vi "AC Voltage Configure.vi"(7 "ChannelList":string, 8 "error in (no error)":errorcluster {"code" format="%.0x"}, 9 "Resolution":dbl, 10 "Range":dbl, 11 "instrument handle":refnum<k15>) -> (0 "error out":errorcluster {"code" format="%.0x"}, 3 "instrument handle out":refnum<k15>)   [LabVIEW 2020, in "Keysight DAQ970.lvlib"]
doc: "Configure the specified channels for AC voltage measurement but does not initiate a scan. This command redefines the scan list."
uses:
  Keysight DAQ970.lvlib
  KtDAQ970.dll
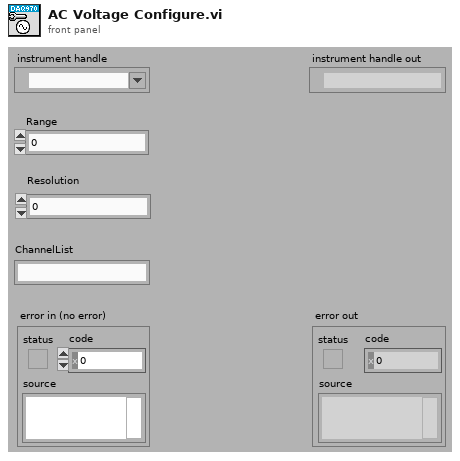
[diagram p1: front panel]
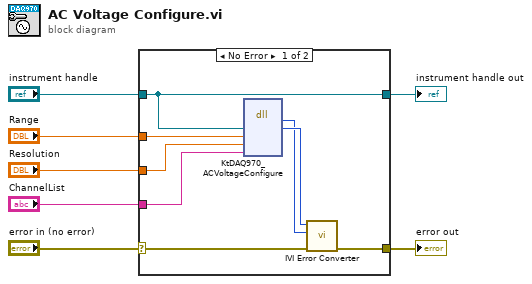
[diagram p0: block diagram]
diagram:
  n1 = case shown="No Error" "error in (no error)" {
    selector: "error in (no error)" -> [w13 w17]
    tunnel: [w12 w17] -> w7
    tunnel: "instrument handle" -> [w8 w16]
    tunnel: "Range" -> [w11 _]
    tunnel: "Resolution" -> [w10 _]
    tunnel: "ChannelList" -> [w9 _]
    tunnel: [w8 w16] -> w1
    frame No Error {
      n2 = dll-call lib="KtDAQ970**.dll" fn="KtDAQ970_ACVoltageConfigure"("Vi"=w8, "Range"=w11, "Resolution"=w10, "ChannelList"=w9) -> (w14:i32, "Vi"=w15:u32)  [unwired: 6 in, 2 out]
      n3 = call "IVI Error Converter.vi"("error in (no error)"=w13, "IVI error code (0)"=w14, "instrument handle"=w15) -> ("error out"=w12:errorcluster)  [unwired: 7 in, 1 out]
    }
    frame Error {
    }
  }
  "error out" <- w7
  "instrument handle out" <- w1
